vi "write read back default.vi"(4 "error in (no error)":errorcluster, 5 "Input Command":string, 6 "Timeout Limit":dbl format="%.2f", 7 "Port Number":refnum<visa-resource-name>) -> (0 "error out":errorcluster, 1 "Timeout":bool, 2 "Query Result":string, 3 "Status Byte":string)   [LabVIEW 2019]
uses:
  Serial Support VISA.llb/Serial Actions.ctl
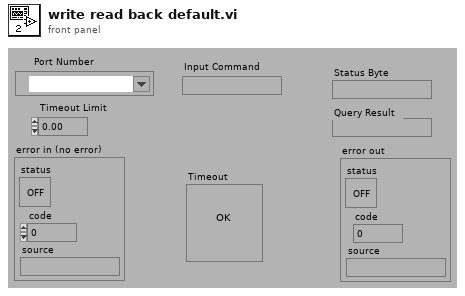
[diagram p1: front panel]
types:
  T1 = typedef "Serial Actions.ctl" = enum16{"Init", "Break", "Clear Buffer", "Write", "Read", "N Bytes", "Lock", "Unlock", "Close"}
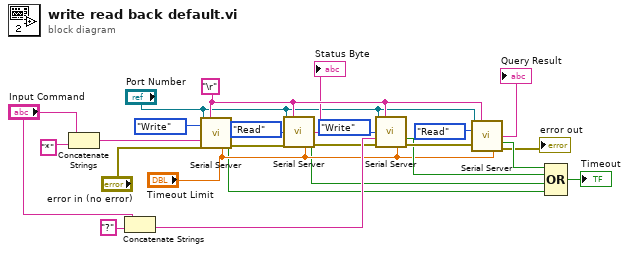
[diagram p0: block diagram]
diagram:
  w15 = "\r" ("EOT Chars (cr/lf)")
  n1 = Concatenate Strings("Input Command", "*" ("Input Command")) -> (w19:string)
  n2 = Concatenate Strings("Input Command", "?") -> (w17:string)
  n3 = call "Serial Server.vi"("VISA Resource Name"="Port Number", "EOT Chars (cr/lf)"=w15, "Action"=Serial_Actions."Write", "String To Send"=w19, "error in (no error)"="error in (no error)", "Timeout Limit(sec)"="Timeout Limit") -> ("Timeout"=w13:bool, "error out"=w10:errorcluster)  [unwired: 5 in, 3 out]
  n4 = call "Serial Server.vi"("VISA Resource Name"="Port Number", "EOT Chars (cr/lf)"=w15, "Action"=Serial_Actions."Read", "error in (no error)"=w10, "Timeout Limit(sec)"="Timeout Limit") -> ("Serial Read"=→"Status Byte":string, "Timeout"=w12:bool, "error out"=w9:errorcluster)  [unwired: 6 in, 2 out]
  n5 = call "Serial Server.vi"("VISA Resource Name"="Port Number", "EOT Chars (cr/lf)"=w15, "Action"=Serial_Actions."Write", "String To Send"=w17, "error in (no error)"=w9, "Timeout Limit(sec)"="Timeout Limit") -> ("Timeout"=w23:bool, "error out"=w24:errorcluster)  [unwired: 5 in, 3 out]
  n6 = call "Serial Server.vi"("VISA Resource Name"="Port Number", "EOT Chars (cr/lf)"=w15, "Action"=Serial_Actions."Read", "error in (no error)"=w24, "Timeout Limit(sec)"="Timeout Limit") -> ("Serial Read"=→"Query Result":string, "Timeout"=w22:bool, "error out"=→"error out":errorcluster)  [unwired: 6 in, 2 out]
  n7 = Compound Arithmetic op=OR(w22, w23, w12, w13) -> (→"Timeout":bool)
